vi "Timestamp with Error.vi"(8 "error in (no error)":errorcluster) -> (0 "error out":errorcluster, 3 "Timestamp":timestamp)   [LabVIEW 2021]
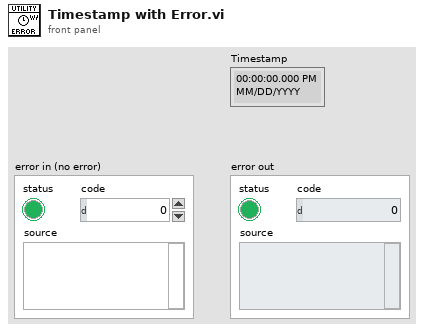
[diagram p1: front panel]
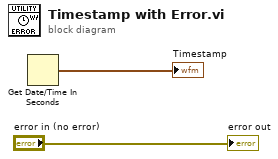
[diagram p0: block diagram]
diagram:
  n1 = Get Date/Time In Seconds() -> (seconds since 1Jan1904=→"Timestamp":timestamp)
  "error out" <- "error in (no error)"
